vi "Temp_Read.vi"(8 "error in (no error)":errorcluster, 9 "Stop Temperature":bool, 11 "reference in":refnum<class "Temp.lvclass">) -> (0 "error out":errorcluster, 3 "reference out":refnum<class "Temp.lvclass">)   [LabVIEW 2017, in "Temp.lvclass"]
uses:
  Temp.lvclass
panel:
  # "This VI is called Asynchronously and will have one instance in memory\nfor each asynchronous call."
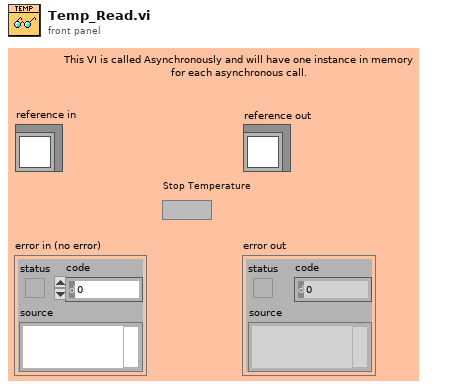
[diagram p1: front panel]
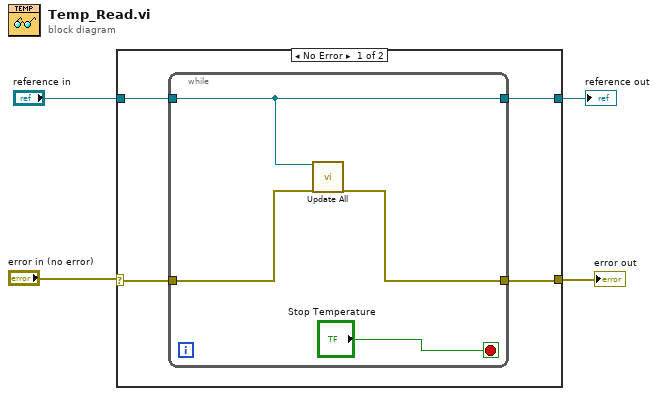
[diagram p0: block diagram]
diagram:
  n1 = case shown="No Error" "error in (no error)" {
    selector: "error in (no error)" -> [w5 w14]
    tunnel: "reference in" -> [w7 w13]
    tunnel: [w8 w13] -> w3
    tunnel: [w6 w14] -> w1
    frame No Error {
      n2 = while {
        tunnel: [w11] -> w8
        tunnel: w7 -> [w11]
        tunnel: [w9] -> w6
        tunnel: w5 -> [w10]
        stop <- "Stop Temperature" stop-if-true
        n3 = call-dynamic "Update All.vi"("reference in"=w11, "error in (no error)"=w10) -> ("error out"=w9:errorcluster)  [unwired: 16 in, 1 out]
      }
    }
    frame Error {
    }
  }
  "error out" <- w1
  "reference out" <- w3
